vi "Read SHV.vi"(8 "error in":errorcluster, 11 "Interlock in":refnum<class "Interlock.lvclass">) -> (0 "error out":errorcluster, 2 "SHV":refnum<k21>, 3 "Interlock out":refnum<class "Interlock.lvclass">)   [LabVIEW 2015, in "Interlocks.lvlib" / "Interlock.lvclass"]
uses:
  Interlock.lvclass
  Interlock.lvclass/Interlock.ctl
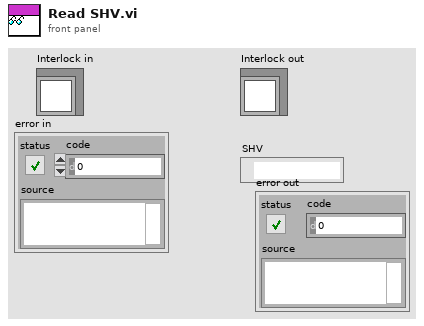
[diagram p1: front panel]
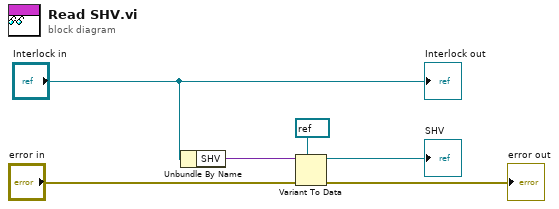
[diagram p0: block diagram]
diagram:
  n1 = Unbundle By Name("Interlock in") -> ("SHV"=w5:variant)
  n2 = Variant To Data(error in="error in", type=refnum<k21> refnum ("SHV"), Variant=w5) -> (data=→"SHV":refnum<k21>, error out=→"error out":errorcluster)
  "Interlock out" <- "Interlock in"
